vi "UpdateLimsTestStepValues.vi"(7 "step_id":u32, 8 "error in (no error)":errorcluster, 9 "duration_hours":dbl, 10 "value":dbl, 11 "ByteGSAPIBase in":refnum<class "ByteGSAPIBase.lvclass">) -> (0 "error out":errorcluster, 2 "Result Step":T1, 3 "ByteGSAPIBase out":refnum<class "ByteGSAPIBase.lvclass">)   [LabVIEW 2019, in "ByteGSWebAPI.lvlib" / "ByteGSAPIBase.lvclass"]
doc: "Carica i dati dello step e ne ritorna il risulato"
uses:
  ByteGSAPIBase.lvclass
  TypeDef/UpdateLimsTestStepData.ctl
  ByteGSAPIBase.lvclass/ByteGSAPIBase.ctl
  <vilib>/Bytelabs/ByteREST/ByteRESTClass/ByteRESTBase/RESTBase.lvclass
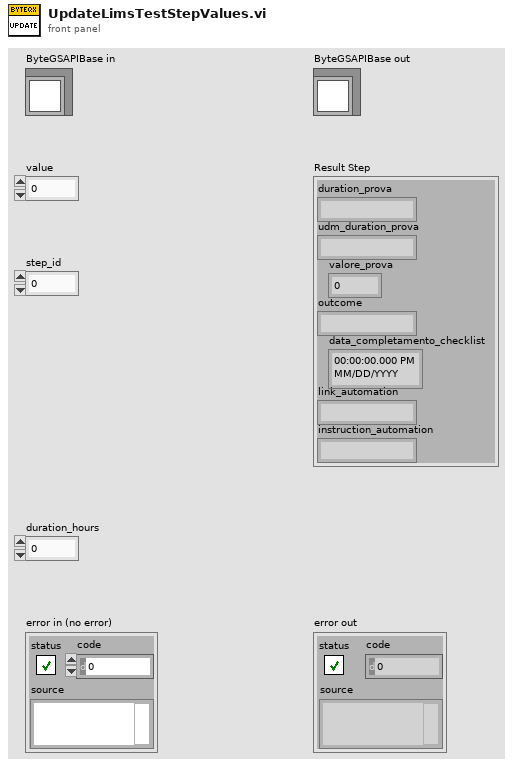
[diagram p1: front panel]
types:
  T1 = typedef "UpdateLimsTestStepData.ctl" = cluster{"duration_prova":string, "udm_duration_prova":string, "valore_prova":dbl, "outcome":string, "data_completamento_checklist":timestamp, "link_automation":string, "instruction_automation":string}
  T2 = cluster{"duration_prova":string, "udm_duration_prova":string, "valore_prova":dbl, "outcome":string, "data_completamento_checklist":timestamp, "link_automation":string, "instruction_automation":string}
  T3 = cluster{"duration_prova":string, "udm_duration_prova":string, "data_completamento_checklist":string, "valore_prova":dbl, "outcome":string, "link_automation":string, "instruction_automation":string}
  T4 = typedef "ByteGSWebAPI.lvlib/ByteGSAPIBase.lvclass/Step.ctl" = cluster{"id":i32, "descrizione":string, "prova":string, "assets":T5[], "criterio_accettazione":string, "valore_criterio_accettazione_max":dbl, "valore_criterio_accettazione_min":dbl, "udm_criterio_accettazione":string, "duration_prova":string, "udm_duration_prova":string, "valore_prova":dbl, "outcome":string, "ordine":i32, "user":i32, "link_automation":string, "instruction_automation":string, "data_completamento_checklist":timestamp}
  T5 = typedef "ByteGSWebAPI.lvlib/ByteGSAPIBase.lvclass/Asset.ctl" = cluster{"descrizione":string, "slug":string, "id":i32}
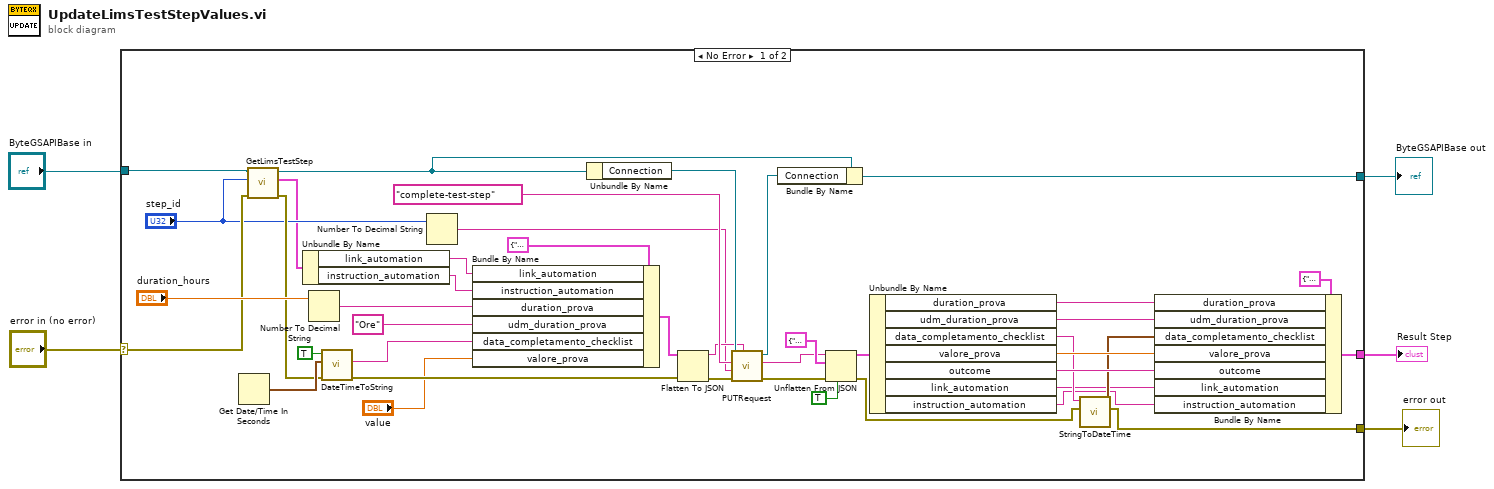
[diagram p0: block diagram]
diagram:
  n1 = case shown="No Error" "error in (no error)" {
    selector: "error in (no error)" -> [w11 w49]
    tunnel: [w20 w49] -> w4
    tunnel: [w46 w48] -> w2
    tunnel: "ByteGSAPIBase in" -> [w13 w48]
    tunnel: [w21 _] -> w1
    frame No Error {
      n2 = Get Date/Time In Seconds() -> (seconds since 1Jan1904=w15:timestamp)
      n3 = call-dynamic "GetLimsTestStep.vi"("error in (no error)"=w11, "Step-id"="step_id", "ByteGSAPIBase in"=w13) -> ("error out"=w10:errorcluster, "StepList"=w8:T4, "ByteGSAPIBase out"=w12:refnum<class "ByteGSAPIBase.lvclass">)  [unwired: 6 in]
      n4 = Unbundle By Name(w8) -> ("link_automation"=w7:string, "instruction_automation"=w6:string)
      n5 = Number To Decimal String(number="duration_hours") -> (decimal integer string=w40:string)  [unwired: 1 in]
      n6 = call "DateTimeToString.vi"("error in"=w10, "current time"=w15, "Time"=TRUE) -> ("error out"=w37:errorcluster, "Date string"=w38:string)  [unwired: 7 in]
      n7 = Number To Decimal String(number="step_id") -> (decimal integer string=w18:string)  [unwired: 1 in]
      n8 = Bundle By Name(cluster=T3 {"duration_prova"="3", "udm_duration_prova"="Ore", "data_completamento_checklist"="2024-10-24T17:19:12Z", "valore_prova"=5.0, "outcome"="P", "link_automation"="", "instruction_automation"=""} ("Update Step"), "link_automation"=w7, "instruction_automation"=w6, "duration_prova"=w40, "udm_duration_prova"="Ore", "data_completamento_checklist"=w38, "valore_prova"="value") -> (w39:T3)
      n9 = Unbundle By Name(w12) -> ("Connection"=w47:refnum<class "RESTBase.lvclass">)
      n10 = Flatten To JSON(anything=w39, error in (no error)=w37) -> (JSON string=w43:string, 11:w42:errorcluster)  [unwired: 1 in]
      n11 = call-dynamic "PUTRequest.vi"("Body in"=w43, "error in (no error)"=w42, "Parameter"=w18, "Request"="complete-test-step", "ByteRESTBase in"=w47) -> ("error out"=w23:errorcluster, "Body"=w22:string, "ByteRESTBase out"=w45:refnum<class "RESTBase.lvclass">)  [unwired: 3 in, 1 out]
      n12 = Bundle By Name(cluster=w12, "Connection"=w45) -> (w46:refnum<class "ByteGSAPIBase.lvclass">)
      n13 = Unflatten From JSON(JSON string=w22, type and defaults=T3 {"duration_prova"="", "udm_duration_prova"="", "data_completamento_checklist"="", "valore_prova"=0.0, "outcome"="P", "link_automation"="", "instruction_automation"=""}, default null elements? (F)=TRUE, error in (no error)=w23) -> (value=w34:T3, error out=w26:errorcluster)  [unwired: 3 in]
      n14 = Unbundle By Name(w34) -> ("duration_prova"=w32:string, "udm_duration_prova"=w31:string, "data_completamento_checklist"=w28:string, "valore_prova"=w30:dbl, "outcome"=w29:string, "link_automation"=w25:string, "instruction_automation"=w24:string)
      n15 = call "StringToDateTime.vi"("error in (no error)"=w26, "datetime string"=w28) -> ("error out"=w20:errorcluster, "timestamp"=w27:timestamp)  [unwired: 8 in]
      n16 = Bundle By Name(cluster=T2 {"duration_prova"="", "udm_duration_prova"="", "valore_prova"=0.0, "outcome"="P", "data_completamento_checklist"=timestamp(0 s since 1904-01-01), "link_automation"="", "instruction_automation"=""}, "duration_prova"=w32, "udm_duration_prova"=w31, "data_completamento_checklist"=w27, "valore_prova"=w30, "outcome"=w29, "link_automation"=w25, "instruction_automation"=w24) -> (w21:T2)
    }
    frame Error {
    }
  }
  "error out" <- w4
  "ByteGSAPIBase out" <- w2
  "Result Step" <- w1
